vi "Write next.vi"(8 "error in (no error)":errorcluster, 10 "next":refnum<data-value>, 11 "Node in":refnum<class "DoublyNode.lvclass">) -> (0 "error out":errorcluster, 3 "Node out":refnum<class "DoublyNode.lvclass">)   [LabVIEW 2021, in "DoublyNode.lvclass"]
uses:
  DoublyNode.lvclass
  IDoublyNode/IDoublyNode.lvclass
  DoublyNode.lvclass/DoublyNode.ctl
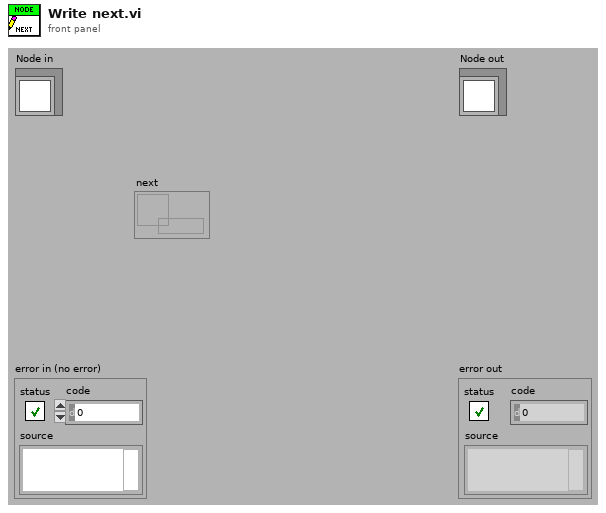
[diagram p1: front panel]
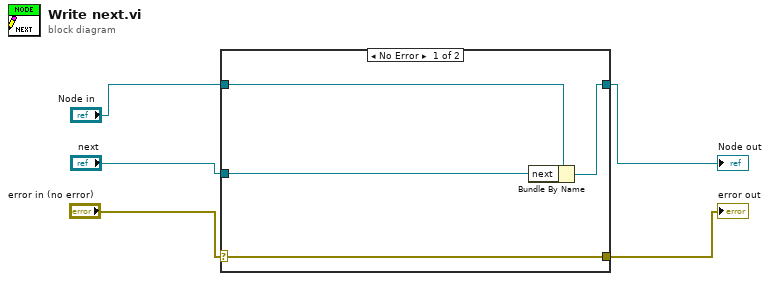
[diagram p0: block diagram]
diagram:
  n1 = case shown="No Error" "error in (no error)" {
    selector: "error in (no error)" -> [w9 w10]
    tunnel: [w9 w10] -> w2
    tunnel: [w7 w11] -> w1
    tunnel: "Node in" -> [w8 w11]
    tunnel: "next" -> [w6 _]
    frame No Error {
      n2 = Bundle By Name(cluster=w8, "next"=w6) -> (w7:refnum<class "DoublyNode.lvclass">)
    }
    frame Error {
    }
  }
  "error out" <- w2
  "Node out" <- w1
